vi "SetAllDigitalOutputs.vi"(4 "error in (no error)":errorcluster, 6 "digital outputs":T1, 7 "axis in":cluster{"keyHandle":u32, "nodeId":u16}={"keyHandle"=0, "nodeId"=1}) -> (0 "error out":errorcluster, 3 "axis out":cluster{"keyHandle":u32, "nodeId":u16}={"keyHandle"=0, "nodeId"=1})   [LabVIEW 2017, in "maxonEPOS.lvlib"]
doc: "<B>SetAllDigitalOutputs</B> writes the state of all digital outputs to the device."
uses:
  Examples/maxonEPOS.lvlib
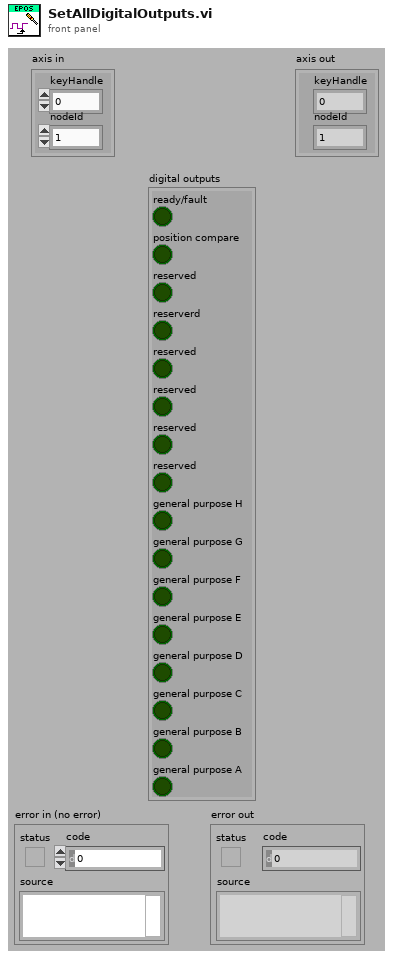
[diagram p1: front panel]
types:
  T1 = cluster{"ready/fault":bool, "position compare":bool, "reserved":bool, "reserverd":bool, "reserved":bool, "reserved":bool, "reserved":bool, "reserved":bool, "general purpose H":bool, "general purpose G":bool, "general purpose F":bool, "general purpose E":bool, "general purpose D":bool, "general purpose C":bool, "general purpose B":bool, "general purpose A":bool}
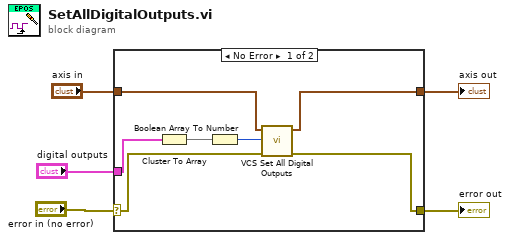
[diagram p0: block diagram]
diagram:
  n1 = case shown="No Error" "error in (no error)" {
    selector: "error in (no error)" -> [w12 w14]
    tunnel: [w9 w14] -> w4
    tunnel: [w10 w13] -> w3
    tunnel: "axis in" -> [w11 w13]
    tunnel: "digital outputs" -> [w6 _]
    frame No Error {
      n2 = Cluster To Array(cluster=w6) -> (array=w7:bool[])
      n3 = Boolean Array To Number(Boolean array=w7) -> (number=w8:u32)
      n4 = call "VCS Set All Digital Outputs.vi"("error in (no error)"=w12, "outputs"=w8, "axis in"=w11) -> ("error out"=w9:errorcluster, "axis out"=w10:cluster{"keyHandle":u32, "nodeId":u16})  [unwired: 7 in]
    }
    frame Error {
    }
  }
  "error out" <- w4
  "axis out" <- w3
